vi "Req Client 2.vi"() -> ()   [LabVIEW 2019, in "RemoteControl.ZMQ.lvclass"]
uses:
  RemoteControl.ZMQ.lvclass
panel:
  in  "stop":bool
  out "Command Sent":string
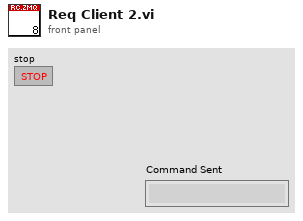
[diagram p1: front panel]
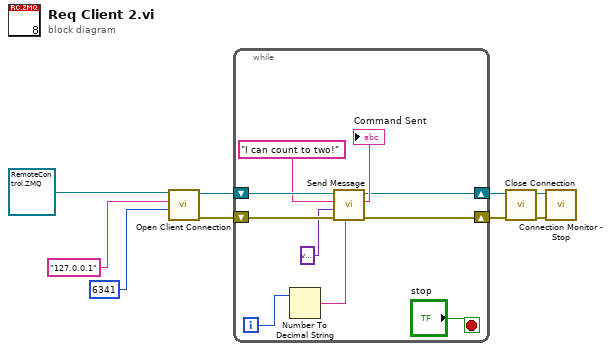
[diagram p0: block diagram]
diagram:
  n1 = call-dynamic "Open Client Connection.vi"("Port"=u16 6341, "address"="127.0.0.1" ("Address"), "RemoteControl.ZMQ in"=refnum<class "RemoteControl.ZMQ.lvclass"> refnum ("RemoteControl.ZMQ.lvclass")) -> ("error out"=w8:errorcluster, "RemoteControl.ZMQ out"=w9:refnum<class "RemoteControl.ZMQ.lvclass">)  [unwired: 7 in]
  n2 = while {
    shift-right: [w14] -> w5
    shift-left: w9 -> [w19]
    shift-right: [w13] -> w4
    shift-left: w8 -> [w18]
    i -> [w12]
    stop <- "stop" stop-if-true
    n3 = Number To Decimal String(number=w12) -> (decimal integer string=w10:string)  [unwired: 1 in]
    n4 = call-dynamic "Send Message.vi"("ID"=w10, "error in (no error)"=w18, "Data"=variant, "Command"="I can count to two!", "RemoteControl.ZMQ in"=w19) -> ("error out"=w13:errorcluster, "ACK"=→"Command Sent":string, "RemoteControl.ZMQ out"=w14:refnum<class "RemoteControl.ZMQ.lvclass">)  [unwired: 4 in]
  }
  n5 = call-dynamic "Close Connection.vi"("error in (no error)"=w4, "RemoteControl.ZMQ in"=w5) -> ("error out"=w6:errorcluster, "RemoteControl.ZMQ out"=w7:refnum<class "RemoteControl.ZMQ.lvclass">)  [unwired: 8 in]
  n6 = call-dynamic "Connection Monitor - Stop.vi"("error in (no error)"=w6, "RemoteControl.ZMQ in"=w7) -> ()  [unwired: 8 in, 2 out]
